vi "TestDAQAIInit.vi"(4 "ConfigData":string, 5 "DAQName":string) -> (0 "Parameter OK":bool, 1 "DAQData":T1, 2 "VI Refnum":refnum<vi>)   [LabVIEW 2020]
uses:
  <vilib>/DAQmx/create/channels.llb/DAQmx Create Channel (AI-Voltage-Basic).vi
  <vilib>/DAQmx/configure/timing.llb/DAQmx Timing (Sample Clock).vi
  <resource>/objmgr/daqmx.rc
panel:
  out "IO":string
  out "InitOK?":bool
  in  "DAQTask":refnum<k21>
  in  "INTYPE":i32(ring)=-1 items=["Default"=-1, "RSE"=10083, "NRSE"=10078, "Differential"=10106, "Pseudodifferential"=12529]
  in  "SPS":dbl
  in  "Len":dbl
  in  "Min":dbl
  in  "Max":dbl
  in  "CH":string
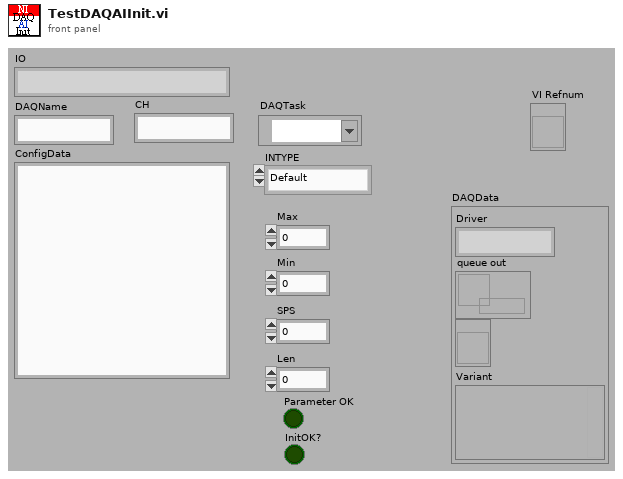
[diagram p1: front panel]
types:
  T1 = cluster{"Driver":string, "queue out":refnum<queue>, refnum<vi>, "Variant":variant}
  T2 = cluster{"Command":string, "Parameter":string, "queue out":refnum<queue>}
  T3 = cluster{"DAQTask":refnum<k21>, "DAQName":string, "CH":string, "Max":dbl, "Min":dbl, "SPS":dbl, "Len":dbl}
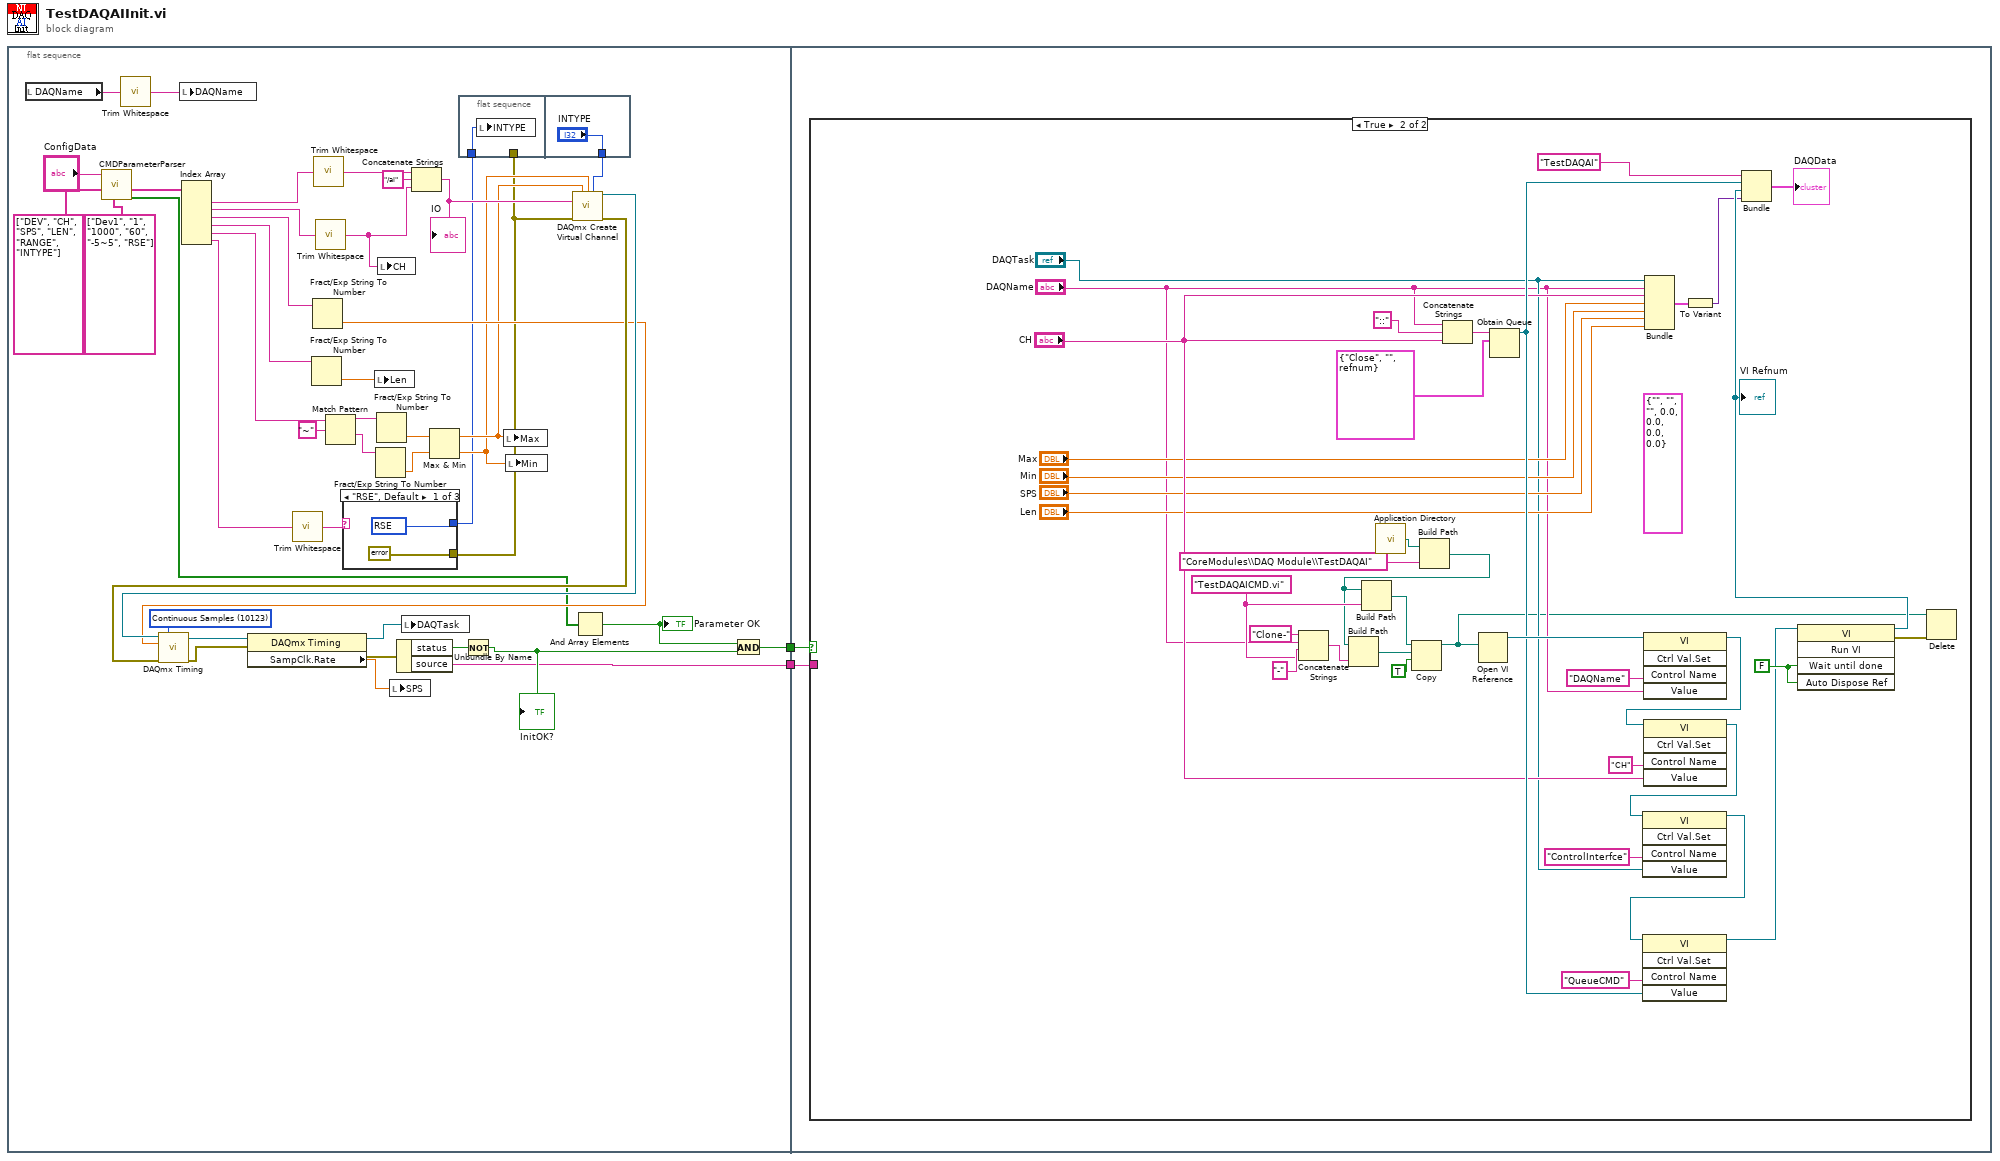
[diagram p0: block diagram]
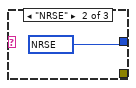
[diagram p2: hidden frame]
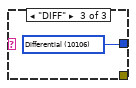
[diagram p3: hidden frame]
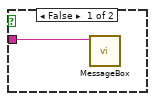
[diagram p4: hidden frame]
diagram:
  n1 = flat-sequence {
    tunnel: [w26] -> w2
    tunnel: [w15] -> w1
    tunnel: w2 -> [w53]
    tunnel: w1 -> [w52]
    frame #0 {
      w24 = 10123 items=["Finite Samples"=10178, "Continuous Samples"=10123, "Hardware Timed Single Point"=12522] ("sample mode")
      n2 = local read "DAQName"() -> (w27:string)
      n3 = call "CMDParameterParser.vi"("DeafultValues"=string[] ["Dev1", "1", "1000", "60", "-5~5", "RSE"] ("ParameterKey"), "RequiredKeys"=string[] ["DEV", "CH", "SPS", "LEN", "RANGE", "INTYPE"] ("ParameterKey"), "CMDParameter"="ConfigData") -> ("KeyFind?"=w3:bool[], "KeyValues"=w11:string[])  [unwired: 6 in, 1 out]
      n4 = call <vilib>:"Trim Whitespace.vi"("string"=w27) -> ("trimmed string"=w28:string)  [unwired: 1 in]
      n5 = local write "DAQName"(w28) -> ()
      n6 = Index Array(array=w11) -> (element #1=w10:string, element #2=w9:string, element #3=w8:string, element #4=w7:string, element #5=w6:string, element #6=w5:string)  [unwired: 6 in]
      n7 = call <vilib>:"Trim Whitespace.vi"("string"=w5) -> ("trimmed string"=w19:string)  [unwired: 1 in]
      n8 = Fract/Exp String To Number(string=w7) -> (number=w42:dbl)  [unwired: 3 in, 1 out]
      n9 = Fract/Exp String To Number(string=w8) -> (number=w35:dbl)  [unwired: 3 in, 1 out]
      n10 = call <vilib>:"Trim Whitespace.vi"("string"=w10) -> ("trimmed string"=w41:string)  [unwired: 1 in]
      n11 = call <vilib>:"Trim Whitespace.vi"("string"=w9) -> ("trimmed string"=w39:string)  [unwired: 1 in]
      n12 = Match Pattern(string=w6, regular expression="~") -> (before substring=w44:string, after substring=w43:string)  [unwired: 1 in, 2 out]
      n13 = case shown="\"RSE\", Default" w19 {
        tunnel: [errorcluster {"status"=FALSE, "code"=0, "source"=""} ("error out") _ _] -> w17
        tunnel: [w49 w50 w51] -> w16
        frame "RSE", Default {
          w49 = 10083 items=["Default"=-1, "RSE"=10083, "NRSE"=10078, "Differential"=10106, "Pseudodifferential"=12529] ("input terminal configuration 2")
        }
        frame "NRSE" {
          w50 = 10078 items=["Default"=-1, "RSE"=10083, "NRSE"=10078, "Differential"=10106, "Pseudodifferential"=12529] ("input terminal configuration 2")
        }
        frame "DIFF" {
          w51 = 10106 items=["Default"=-1, "RSE"=10083, "NRSE"=10078, "Differential"=10106, "Pseudodifferential"=12529] ("input terminal configuration 2")
        }
      }
      n14 = local write "Len"(w42) -> ()
      n15 = Fract/Exp String To Number(string=w43) -> (number=w22:dbl)  [unwired: 3 in, 1 out]
      n16 = Fract/Exp String To Number(string=w44) -> (number=w23:dbl)  [unwired: 3 in, 1 out]
      n17 = local write "CH"(w39) -> ()
      n18 = Concatenate Strings(w41, "/ai" ("string"), w39) -> (w38:string)
      "IO" <- w38
      n19 = Max & Min(x=w23, y=w22) -> (max(x,y)=w21:dbl, min(x,y)=w20:dbl)
      n20 = flat-sequence {
        tunnel: w17 -> [_]
        tunnel: w16 -> [w46]
        tunnel: ["INTYPE"] -> w18
        frame #0 {
          n21 = local write "INTYPE"(w46) -> ()
        }
        frame #1 {
        }
      }
      n22 = local write "Max"(w21) -> ()
      n23 = local write "Min"(w20) -> ()
      n24 = call-poly <vilib>:"DAQmx Create Virtual Channel.vi"("maximum value"=w21, "minimum value"=w20, "input terminal configuration"=w18, "physical channels"=w38, "error in"=w17) -> ("task out"=w36:refnum<k21>, "error out"=w37:errorcluster)  [unwired: 9 in]
      n25 = call-poly <vilib>:"DAQmx Timing.vi"("task/channels in"=w36, "sample mode"=w24, "rate"=w35, "error in"=w37) -> ("task out"=w34:refnum<k21>, "error out"=w33:errorcluster)  [unwired: 10 in]
      n26 = property class="DAQmx Timing"(reference=w34, error in=w33) -> (reference out=w29:refnum<k21>, error out=w31:errorcluster, "SampClk.Rate"=w32:dbl)
      n27 = local write "SPS"(w32) -> ()
      n28 = Unbundle By Name(w31) -> ("status"=w30:bool, "source"=w15:string)
      n29 = local write "DAQTask"(w29) -> ()
      n30 = Not(x=w30) -> (.not. x?=w25:bool)
      "InitOK?" <- w25
      n31 = And Array Elements(Boolean array=w3) -> (logical AND=w4:bool)
      "Parameter OK" <- w4
      n32 = And(x=w4, y=w25) -> (x .and. y?=w26:bool)
    }
    frame #1 {
      n33 = case shown="True" w53 {
        tunnel: w52 -> [w54 _]
        frame False {
          n34 = call "MessageBox.vi"("!!!!!!!!!!!!!Message!!!!!!!!!!!!!"=w54) -> ()  [unwired: 10 in, 1 out]
        }
        frame True {
          (unwired) T3 {"DAQTask"="", "DAQName"="", "CH"="", "Max"=0.0, "Min"=0.0, "SPS"=0.0, "Len"=0.0} ("output cluster")
          w72 = FALSE ("Wait Until Done")
          w83 = "TestDAQAICMD.vi" ("name or relative path")
          n35 = Concatenate Strings("Clone-" ("string"), "DAQName", "-" ("string"), w83) -> (w87:string)
          n36 = call <vilib>:"Application Directory.vi"() -> ("Application Directory"=w66:path)
          n37 = Build Path(base path=w66, name or relative path="CoreModules\\DAQ Module\\TestDAQAI") -> (appended path=w65:path)
          n38 = Build Path(base path=w65, name or relative path=w87) -> (appended path=w85:path)
          n39 = Build Path(base path=w65, name or relative path=w83) -> (appended path=w82:path)
          n40 = Copy(9:TRUE ("overwrite (F)"), 10:w85, 11:w82) -> (3:w56:path)  [unwired: 2 in, 2 out]
          n41 = Concatenate Strings("DAQName", "::" ("string"), "CH") -> (w91:string)
          n42 = Open VI Reference(vi path=w56) -> (vi reference=w77:refnum<vi>)  [unwired: 5 in, 1 out]
          n43 = Obtain Queue(name (unnamed)=w91, element data type=T2 {"Command"="Close", "Parameter"="", "queue out"=refnum} ("Motor Module CMD")) -> (queue out=w76:refnum<queue>)  [unwired: 3 in, 2 out]
          n44 = invoke class="VI" method="Ctrl Val.Set"(reference=w77, "Control Name"="DAQName", "Value"="DAQName") -> (reference out=w75:refnum<vi>)  [unwired: 2 in, 4 out]
          n45 = invoke class="VI" method="Ctrl Val.Set"(reference=w75, "Control Name"="CH", "Value"="CH") -> (reference out=w74:refnum<vi>)  [unwired: 2 in, 4 out]
          n46 = invoke class="VI" method="Ctrl Val.Set"(reference=w74, "Control Name"="ControlInterfce", "Value"="DAQTask") -> (reference out=w73:refnum<vi>)  [unwired: 2 in, 4 out]
          n47 = invoke class="VI" method="Ctrl Val.Set"(reference=w73, "Control Name"="QueueCMD", "Value"=w76) -> (reference out=w55:refnum<vi>)  [unwired: 2 in, 4 out]
          n48 = Bundle("DAQTask"="DAQTask", "DAQName"="DAQName", "CH"="CH", "Max"="Max", "Min"="Min", "SPS"="SPS", "Len"="Len") -> (w92:T3)  [unwired: 1 in]
          n49 = To Variant(anything=w92) -> (Variant=w69:variant)
          n50 = invoke class="VI" method="Run VI"(reference=w55, "Wait until done"=w72, "Auto Dispose Ref"=w72) -> (reference out=w70:refnum<vi>, error out=w57:errorcluster)  [unwired: 2 in, 3 out]
          "VI Refnum" <- w70
          n51 = Bundle("Driver"="TestDAQAI", "queue out"=w76, w70, "Variant"=w69) -> (→"DAQData":T1)  [unwired: 1 in]
          n52 = Delete(path (use dialog)=w56, error in=w57) -> ()  [unwired: 3 in, 3 out]
        }
      }
    }
  }
